vi "Global - Logging Time.vi"() -> ()   [LabVIEW 2019]
panel:
  in  "Prev Time":dbl
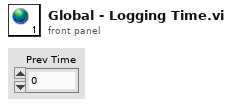
[diagram p1: front panel]
diagram:
